vi "Global - Configuration Options.vi"() -> ()   [LabVIEW 2017]
panel:
  in  "Connected?":bool
  in  "Network Stream Buffer Size":i32=50
  in  "Network Stream Polling Timeout (ms)":i32=500
  in  "RT Stream Name":string="Command Stream from RT"
  in  "UI Stream Name":string="Command Stream from UI"
  in  "Network Stream Connect Timeout (ms)":i32=5000
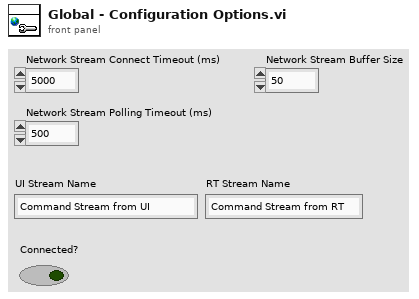
[diagram p1: front panel]
diagram:
